vi "SerialReadSpeedTest.vi"() -> ()   [LabVIEW 2013]
uses:
  <vilib>/Instr/_visa.llb/VISA Configure Serial Port (Instr).vi
panel:
  out "time dt(ms)":dbl
  in  "t2":dbl
  in  "t1":dbl
  out "output_int16":i32[](array[numeric])
  out "unsigned byte array 2":u8[](array[numeric]) caption="unsigned byte array input"
  in  "stop":bool
  in  "serial_port":refnum<visa-resource-name> caption="Porta Serial"
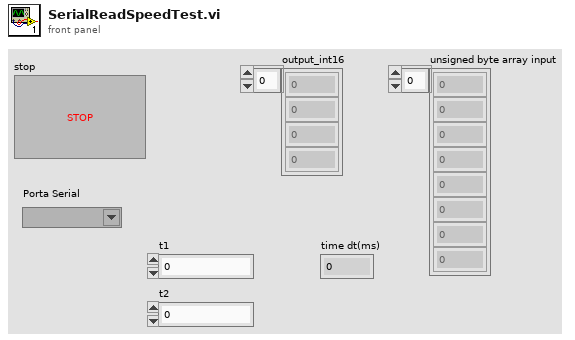
[diagram p1: front panel]
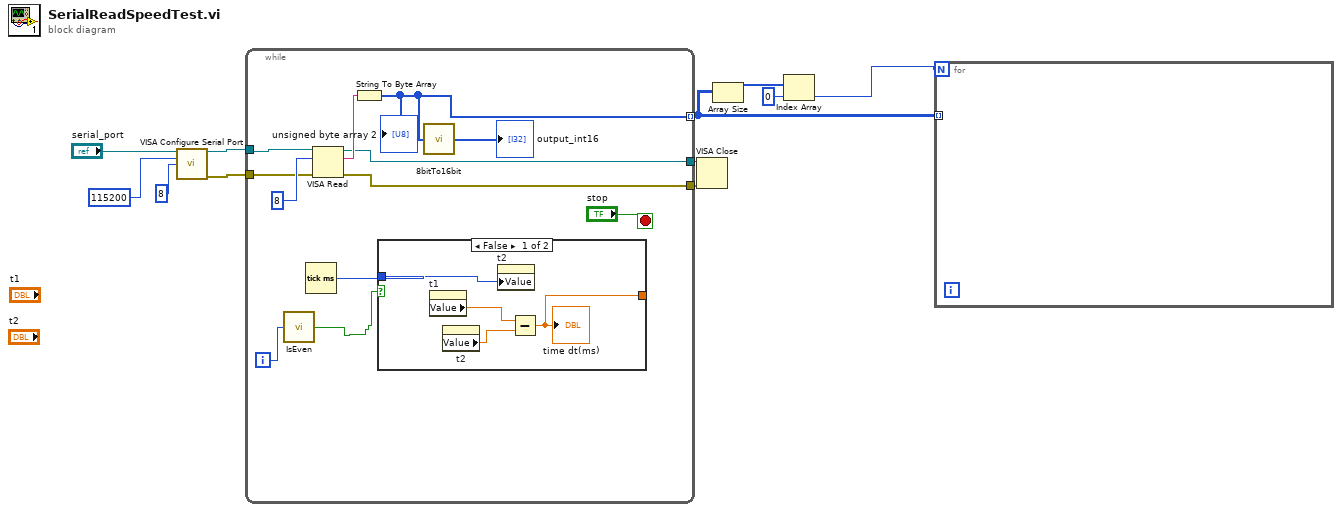
[diagram p0: block diagram]
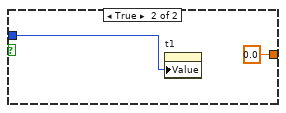
[diagram p2: hidden frame]
diagram:
  n1 = call-poly "VISA Configure Serial Port"("VISA resource name"="serial_port", "baud rate (9600)"=u32 115200, "data bits (8)"=u16 8) -> ("VISA resource name out"=w8:refnum<visa-resource-name>, "error out"=w7:errorcluster)  [unwired: 11 in]
  n2 = while {
    tunnel: w8 -> [w22]
    tunnel: w7 -> [w21]
    tunnel: [w19] -> w6
    tunnel: [w18] -> w5
    tunnel: [w16] -> w4 mode=indexing
    i -> [w13]
    stop <- "stop" stop-if-true
    n3 = call "IsEven.vi"("Numeric"=w13) -> ("Boolean"=w12:bool)
    n4 = Tick Count (ms)() -> (millisecond timer value=w14:u32)
    n5 = VISA Read(VISA resource name=w22, byte count=u32 8, error in (no error)=w21) -> (VISA resource name out=w18:refnum<visa-resource-name>, read buffer=w20:string, error out=w19:errorcluster)  [unwired: 1 out]
    n6 = String To Byte Array(string=w20) -> (unsigned byte array=w16:u8[])
    "unsigned byte array 2" <- w16
    n7 = case shown="False" w12 {
      tunnel: w14 -> [w27 w29]
      tunnel: [w24 0.0] -> _
      frame False {
        n8 = property on="t1" class="DigNum (strict)"() -> ("Value"=w26:dbl)  [unwired: 2 in, 2 out]
        n9 = property on="t2" class="DigNum (strict)"() -> ("Value"=w25:dbl)  [unwired: 2 in, 2 out]
        n10 = property on="t2" class="DigNum (strict)"("Value"=w27) -> ()  [unwired: 2 in, 2 out]
        n11 = Subtract(x=w26, y=w25) -> (x-y=w24:dbl)
        "time dt(ms)" <- w24
      }
      frame True {
        n12 = property on="t1" class="DigNum (strict)"("Value"=w29) -> ()  [unwired: 2 in, 2 out]
      }
    }
    n13 = call "8bitTo16bit.vi"("input_byte"=w16) -> ("output_int16"=→"output_int16":i32[])
  }
  n14 = VISA Close(VISA resource name=w5, error in (no error)=w6) -> ()  [unwired: 1 out]
  n15 = Array Size(array=w4) -> (size(s)=w3:i32[])
  n16 = Index Array(array=w3, index=0) -> (element=w1:i32)
  n17 = for {
    N: w1 -> [_]
    tunnel: w4 -> [_] mode=indexing
  }
